vi "GitCheckoutMasterHead.vi"(8 "error in (no error)":errorcluster, 9 "File":path=path "", 11 "Git exec":string="git") -> (0 "error out":errorcluster, 1 "File out":path, 2 "Response":string, 3 "Git exec out":string="git")   [LabVIEW 2013]
uses:
  GitCmd.vi
  <vilib>/dlg_ctls.llb/Space Constant.vi
  <vilib>/Platform/system.llb/System Exec.vi
  <vilib>/Utility/error.llb/Error Cluster From Error Code.vi
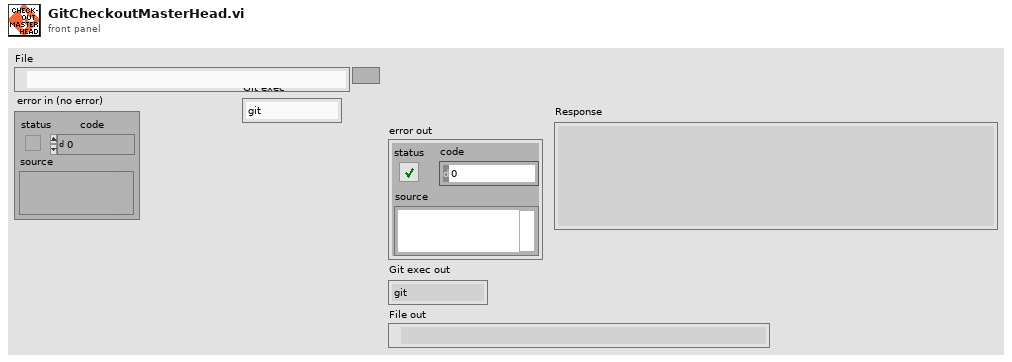
[diagram p1: front panel]
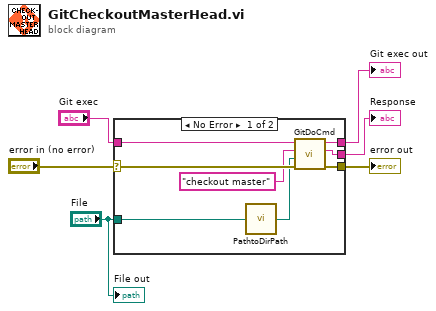
[diagram p0: block diagram]
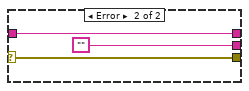
[diagram p2: hidden frame]
diagram:
  n1 = case shown="No Error" "error in (no error)" {
    selector: "error in (no error)" -> [w11 w16]
    tunnel: "Git exec" -> [w14 w15]
    tunnel: "File" -> [w9 _]
    tunnel: [w12 ""] -> w4
    tunnel: [w10 w16] -> w3
    tunnel: [w13 w15] -> w1
    frame No Error {
      n2 = call "PathtoDirPath.vi"("Path"=w9) -> ("Path out"=w8:path)
      n3 = call "GitDoCmd.vi"("error in (no error)"=w11, "Working Path"=w8, "Git command"="checkout master" ("string"), "Git exec"=w14) -> ("error out"=w10:errorcluster, "Returned stdout"=w12:string, "Git exec out"=w13:string)  [unwired: 3 in, 1 out]
    }
    frame Error {
    }
  }
  "Response" <- w4
  "error out" <- w3
  "Git exec out" <- w1
  "File out" <- "File"
